vi "GetAllMatchInfo.vi"(8 "error in (no error)":errorcluster caption="错误输入（无错误）", 9 "pstInfo In":cluster{"nInfoSize":u32, "nType":u32}, 10 "handle":u64, 11 "pInfo":u64[](array[numeric])) -> (0 "error out":errorcluster caption="错误输出", 1 "pstInfo Out":cluster{"nInfoSize":u32, "nType":u32}, 2 "handle out":u64, 3 "function return":i32)   [LabVIEW 2013, in "MvCameraControl.lvlib"]
doc: "MV_LV_API int __stdcall SaveImage(MV_SAVE_IMAGE_PARAM* pSaveParam);"
uses:
  MvCameraControl.lvlib
  MvCameraPatch.dll
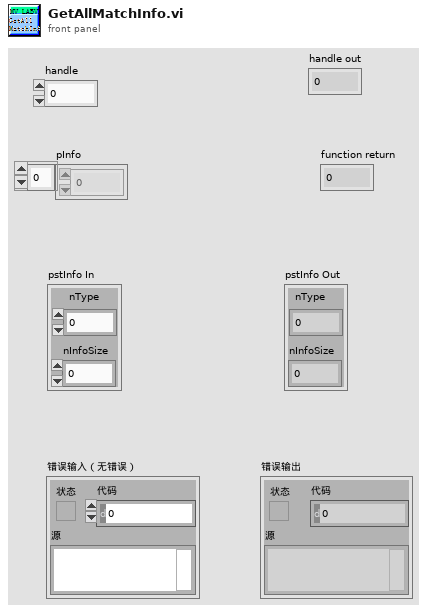
[diagram p1: front panel]
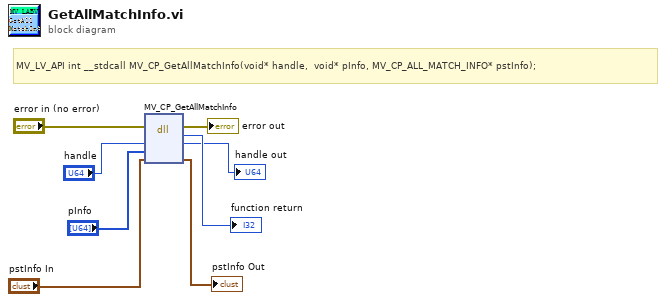
[diagram p0: block diagram]
diagram:
  # "MV_LV_API int __stdcall MV_CP_GetAllMatchInfo(void* handle,  void* pInfo, MV_CP_ALL_MATCH_INFO* pstInfo);"
  n1 = dll-call lib="MvCameraPatch.dll" fn="MV_CP_GetAllMatchInfo"(error in="error in (no error)", "handle"="handle", "pInfo"="pInfo", "pstInfo"="pstInfo In") -> (error out=→"error out":errorcluster, "返回类型"=→"function return":i32, "handle"=→"handle out":u64, "pstInfo"=→"pstInfo Out":cluster{"nInfoSize":u32, "nType":u32})  [unwired: 3 in, 1 out]
